vi "CSV_Setup_Data_Create.vi"(3 "error in (no error)":errorcluster, 4 "Setup Data File":string, 6 "Setup Data path":string) -> (0 "error out":errorcluster, 1 "File Path":string, 2 "Setup Data File path":path)   [LabVIEW 2024]
uses:
  <vilib>/Utility/file.llb/Write Delimited Spreadsheet (string).vi
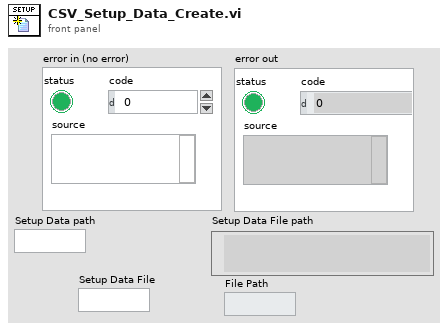
[diagram p1: front panel]
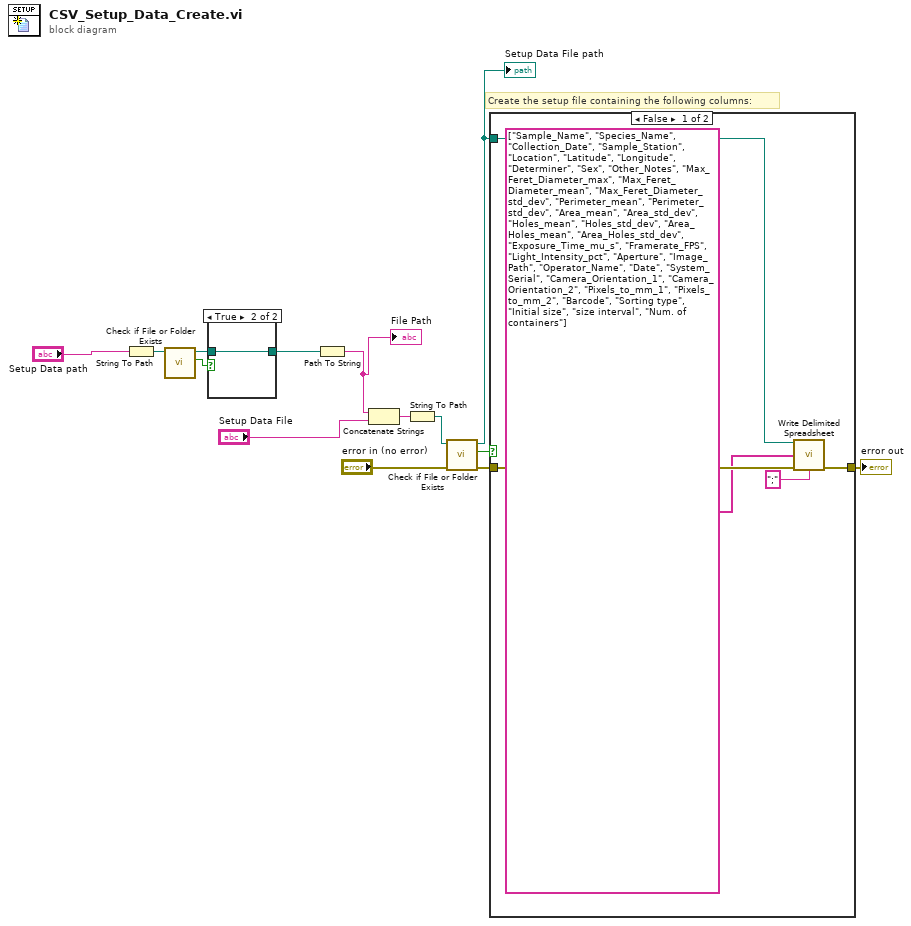
[diagram p0: block diagram]
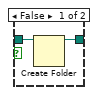
[diagram p2: hidden frame]
diagram:
  # "Create the setup file containing the following columns:"
  n1 = String To Path(string="Setup Data path") -> (path=w7:path)
  n2 = call <vilib>:"Check if File or Folder Exists.vi"("path"=w7) -> ("file or folder exists?"=w6:bool, "dup path"=w5:path)  [unwired: 8 in, 1 out]
  n3 = case shown="True" w6 {
    tunnel: w5 -> [w16 w17]
    tunnel: [w15 w17] -> w4
    frame False {
      n4 = Create Folder(path (use dialog)=w16) -> (created path=w15:path)  [unwired: 2 in, 2 out]
    }
    frame True {
    }
  }
  n5 = Path To String(path=w4) -> (string=w1:string)
  "File Path" <- w1
  n6 = Concatenate Strings(w1, "Setup Data File") -> (w14:string)
  n7 = String To Path(string=w14) -> (path=w13:path)
  n8 = call <vilib>:"Check if File or Folder Exists.vi"("error in (no error)"="error in (no error)", "path"=w13) -> ("error out"=w10:errorcluster, "file or folder exists?"=w12:bool, "dup path"=w11:path)  [unwired: 7 in]
  "Setup Data File path" <- w11
  n9 = case shown="False" w12 {
    tunnel: w11 -> [w21 _]
    tunnel: w10 -> [w20 w23]
    tunnel: [w19 w23] -> w8
    frame False {
      n10 = call-poly <vilib>:"Write Delimited Spreadsheet.vi"("file path (dialog if empty)"=w21, "1D data"=string[] ["Sample_Name", "Species_Name", "Collection_Date", "Sample_Station", "Location", "Latitude", "Longitude", "Determiner", "Sex", "Other_Notes", "Max_Feret_Diameter_max", "Max_Feret_Diameter_mean", "Max_Feret_Diameter_std_dev", "Perimeter_mean", "Perimeter_std_dev", "Area_mean", "Area_std_dev", "Holes_mean", "Holes_std_dev", "Area_Holes_mean", "Area_Holes_std_dev", "Exposure_Time_mu_s", "Framerate_FPS", "Light_Intensity_pct", "Aperture", "Image_Path", "Operator_Name", "Date", "System_Serial", "Camera_Orientation_1", "Camera_Orientation_2", "Pixels_to_mm_1", "Pixels_to_mm_2", "Barcode", "Sorting type", "Initial size", "size interval", "Num. of containers"], "error in (no error)"=w20, "delimiter (\\t)"=";" ("delimiter (\\t)")) -> ("error out"=w19:errorcluster)  [unwired: 10 in, 1 out]
    }
    frame True {
    }
  }
  "error out" <- w8
